vi "Phasor  Explorer SEPL Plot Name.vi"(8 "Error In":errorcluster, 11 "Phasor Parameters":T1 {"Detector Parameters"."Frames/Image" min=1; "Detector Parameters"."Multiplicity" min=0; "Detector Parameters"."Bits/Frame" min=1; "Detector Parameters"."Gates/Frame" min=1; "Gate Parameters"."# Steps" min=0.0; "Gate Parameters"."Tolerance" min=0.0; "Gate Parameters"."Top Slope" min=0.0; "Gate Parameters"."Edge Width" min=0.0; "Gate Parameters"."Gate Step" min=0.0; "Gate Parameters"."# Gates" min=0.0 step=1.0; "Gate Parameters"."Gate Width" min=0.0; "Decay & IRF Parameters"."Lifetime" min=0.0; "Decay & IRF Parameters"."IRF Period" min=0.0; "Phasor Parameters"."Square Gate Width" min=0.0; "Phasor Parameters"."# Gates" min=0.0; "Phasor Parameters"."Calibration Lifetime" min=0.0; "Phasor Parameters"."Harmonic Frequency" min=0.0; "Display Parameters"."Min tau" min=0.0; "Display Parameters"."Max tau" min=0.0; "Display Parameters"."# Points" min=1 step=1}) -> (0 "Error Out":errorcluster, 3 "SEPL Plot Name":string)   [LabVIEW 2019]
uses:
  SEPL Parameters.ctl
  Phasor Explorer Display Parameters.ctl
  Type of Series.ctl
  Phasor Explorer Phasor Parameters.ctl
  Phasor Calculation Type.ctl
  SEPL Type.ctl
  Phasor Explorer Decay Parameters.ctl
  IRF Model.ctl
  Phasor Explorer Gate Parameters.ctl
  Gate Type.ctl
  Type of User-defined Function.ctl
  Phasor Explorer Detector Parameters.ctl
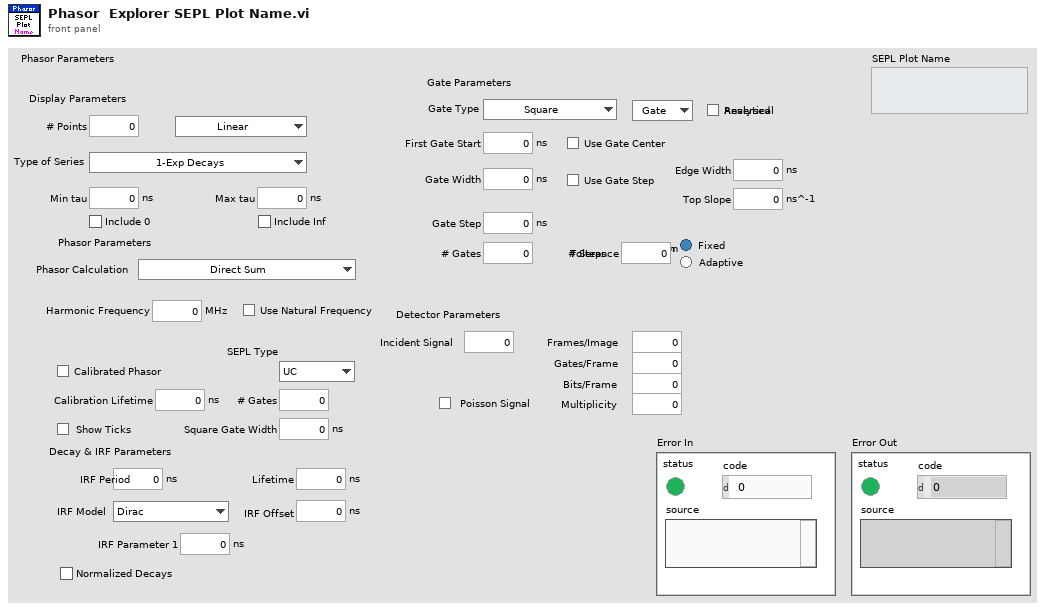
[diagram p1: front panel]
types:
  T1 = typedef "SEPL Parameters.ctl" = cluster{"Display Parameters":T2, "Phasor Parameters":T4, "Decay & IRF Parameters":T7, "Gate Parameters":T9, "Detector Parameters":T12}
  T2 = typedef "Phasor Explorer Display Parameters.ctl" = cluster{"# Points":i32, "Ramp Type":enum16{"Linear", "Logarithmic"}, "Type of Series":T3, "Min tau":dbl[unit], "Max tau":dbl[unit], "Include 0":bool, "Include Infinity":bool}
  T3 = typedef "Type of Series.ctl" = enum16{"1-Exp Decays", "Linear Combination of 1-Exp"}
  T4 = typedef "Phasor Explorer Phasor Parameters.ctl" = cluster{"Harmonic Frequency":dbl[unit], "Use f* = 1/D Frequency":bool, "Calibrated Phasor":bool, "Calibration Lifetime":dbl[unit], "Phasor Calculation":T5, "SEPL Type":T6, "# Gates":dbl, "Square Gate Width":dbl[unit], "Show Ticks":bool}
  T5 = typedef "Phasor Calculation Type.ctl" = enum16{"Direct Sum", "Analytical Formula"}
  T6 = typedef "SEPL Type.ctl" = enum16{"UC", "L_N", "L_N[W]", "L_X"}
  T7 = typedef "Phasor Explorer Decay Parameters.ctl" = cluster{"Lifetime":dbl[unit], "IRF Offset":dbl[unit], "IRF Period":dbl[unit], "Normalized Decays":bool, "IRF Model":T8, "IRF Parameter 1":dbl[unit]}
  T8 = typedef "IRF Model.ctl" = enum16{"Dirac", "Exponential"}
  T9 = typedef "Phasor Explorer Gate Parameters.ctl" = cluster{"First Gate Start":dbl[unit], "Use Gate Center":bool, "Gate Width":dbl[unit], "Gate Step":dbl[unit], "# Gates":dbl, "Gate Type":T10, "Edge Width":dbl[unit], "Top Slope":dbl[unit], "Reversed Sawtooth?":bool, "Analytical Computation":bool, "Integration":enum32{"Item 0", "Item 1"}, "Tolerance":dbl, "# Steps":dbl, "Type of User-defined Function":T11, "Use Gate Step":bool}
  T10 = typedef "Gate Type.ctl" = enum16{"Square", "Finite Edge Square", "Finite Edge, Tilted Top Square", "Triangle", "Sawtooth", "User-defined"}
  T11 = typedef "Type of User-defined Function.ctl" = enum16{"Gate", "IRF"}
  T12 = typedef "Phasor Explorer Detector Parameters.ctl" = cluster{"Frames/Image":i32, "Gates/Frame":i32, "Bits/Frame":i32, "Multiplicity":i32, "Incident Signal":dbl, "Poisson Signal":bool}
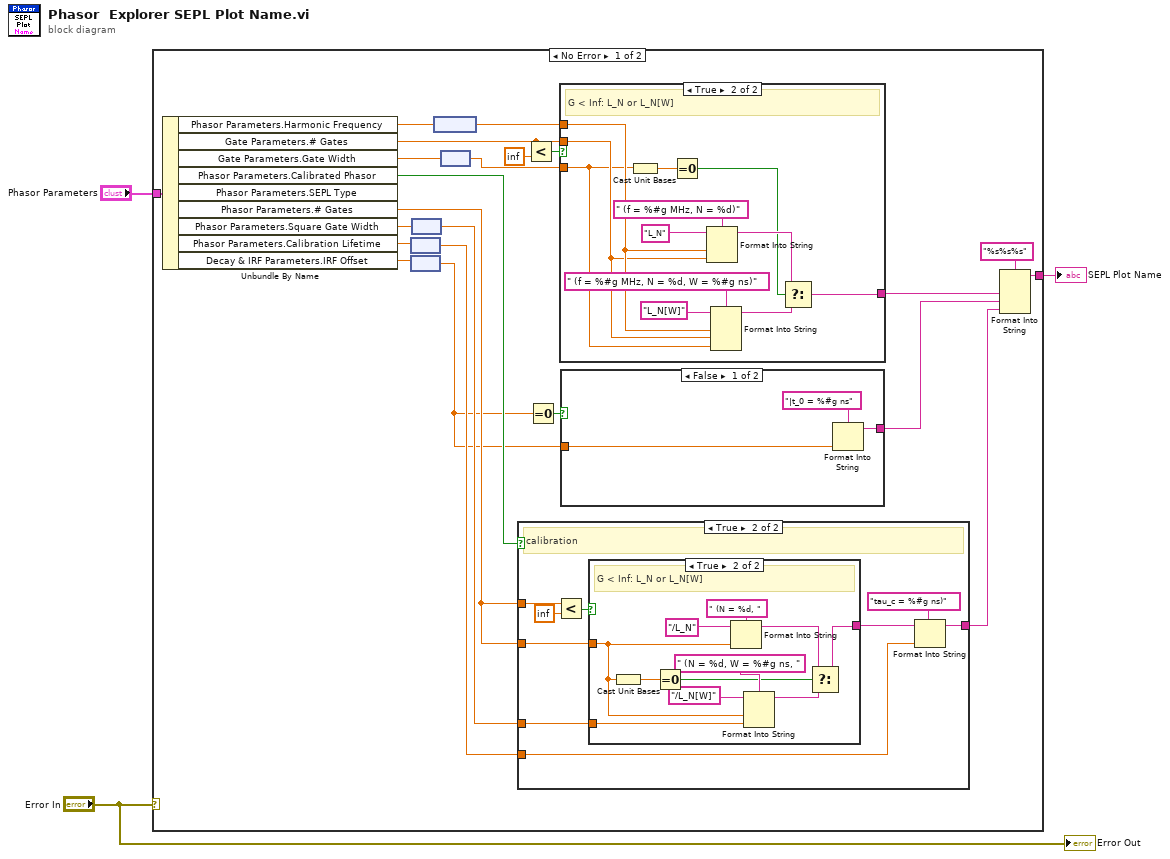
[diagram p0: block diagram]
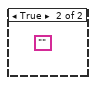
[diagram p2: hidden frame]
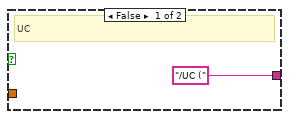
[diagram p4: hidden frame]
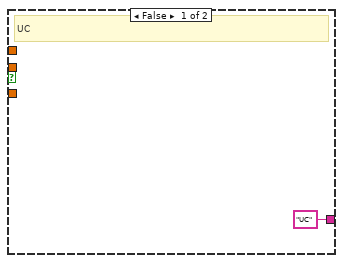
[diagram p5: hidden frame]
diagram:
  n1 = case shown="No Error" "Error In" {
    tunnel: "Phasor Parameters" -> [w24 _]
    tunnel: [w19 _] -> w2
    frame No Error {
      n2 = Unbundle By Name(w24) -> ("Phasor Parameters.Harmonic Frequency"=w18:dbl[unit], "Gate Parameters.# Gates"=w17:dbl, "Gate Parameters.Gate Width"=w16:dbl[unit], "Phasor Parameters.Calibrated Phasor"=w15:bool, "Phasor Parameters.# Gates"=w12:dbl, "Phasor Parameters.Square Gate Width"=w14:dbl[unit], "Phasor Parameters.Calibration Lifetime"=w9:dbl[unit], "Decay & IRF Parameters.IRF Offset"=w7:dbl[unit])  [unwired: 1 out]
      n3 = node(w9) -> (w20:dbl)
      n4 = node(w7) -> (w4:dbl)
      n5 = node(w14) -> (w10:dbl)
      n6 = node(w18) -> (w13:dbl)
      n7 = node(w16) -> (w8:dbl)
      n8 = case shown="True" w15 {
        tunnel: w20 -> [_ w32]
        tunnel: w12 -> [_ w37]
        tunnel: w12 -> [_ w35]
        tunnel: [_ w31] -> w11
        tunnel: w10 -> [_ w29]
        frame False {
          # "no calibration"
        }
        frame True {
          # "calibration"
          n9 = Less?(x=w35, y=inf) -> (x < y?=w34:bool)
          n10 = case shown="True" w34 {
            tunnel: w37 -> [_ w41]
            tunnel: ["/UC (" ("initial string") w39] -> w30
            tunnel: w29 -> [_ w40]
            frame False {
              # "UC"
            }
            frame True {
              # "G < Inf: L_N or L_N[W]"
              n11 = Cast Unit Bases(0:w41) -> (2:w43:dbl)  [unwired: 1 in]
              n12 = Equal To 0?(x=w43) -> (x = 0?=w42:bool)
              n13 = Format Into String(format string=" (N = %d, ", initial string="/L_N" ("t"), w41) -> (resulting string=w47:string)  [unwired: 1 in, 1 out]
              n14 = Format Into String(format string=" (N = %d, W = %#g ns, ", initial string="/L_N[W]" ("f"), w41, w40) -> (resulting string=w44:string)  [unwired: 1 in, 1 out]
              n15 = Select(t=w47, s=w42, f=w44) -> (s? t:f=w39:string)
            }
          }
          n16 = Format Into String(format string="tau_c = %#g ns)", initial string=w30, w32) -> (resulting string=w31:string)  [unwired: 1 in, 1 out]
        }
      }
      n17 = Less?(x=w17, y=inf) -> (x < y?=w23:bool)
      n18 = Equal To 0?(x=w4) -> (x = 0?=w6:bool)
      n19 = case shown="True" w23 {
        tunnel: ["UC" w62] -> w21
        tunnel: w17 -> [_ w54]
        tunnel: w8 -> [_ w52]
        tunnel: w13 -> [_ w55]
        frame False {
          # "UC"
        }
        frame True {
          # "G < Inf: L_N or L_N[W]"
          n20 = Cast Unit Bases(0:w52) -> (2:w53:dbl)  [unwired: 1 in]
          n21 = Equal To 0?(x=w53) -> (x = 0?=w51:bool)
          n22 = Format Into String(format string=" (f = %#g MHz, N = %d)", initial string="L_N" ("t"), w55, w54) -> (resulting string=w59:string)  [unwired: 1 in, 1 out]
          n23 = Format Into String(format string=" (f = %#g MHz, N = %d, W = %#g ns)", initial string="L_N[W]" ("f"), w55, w54, w52) -> (resulting string=w56:string)  [unwired: 1 in, 1 out]
          n24 = Select(t=w59, s=w51, f=w56) -> (s? t:f=w62:string)
        }
      }
      n25 = case shown="False" w6 {
        tunnel: [w28 _] -> w5
        tunnel: w4 -> [w26 _]
        frame False {
          n26 = Format Into String(format string="|t_0 = %#g ns", w26) -> (resulting string=w28:string)  [unwired: 2 in, 1 out]
        }
        frame True {
          (unwired) ""
        }
      }
      n27 = Format Into String(format string="%s%s%s", w21, w5, w11) -> (resulting string=w19:string)  [unwired: 2 in, 1 out]
    }
    frame Error {
    }
  }
  "SEPL Plot Name" <- w2
  "Error Out" <- "Error In"
